vi "Run_Post Core.vi"(0 "For Loop in":refnum<class "While Loop.lvclass">, 11 "error in (no error)":errorcluster) -> (4 "For Loop out":refnum<class "While Loop.lvclass">, 6 "Go to Run Pre Core?":bool, 15 "error out":errorcluster)   [LabVIEW 2016, in "While Loop.lvclass"]
uses:
  While Loop.lvclass
  While Loop.lvclass/While Loop.ctl
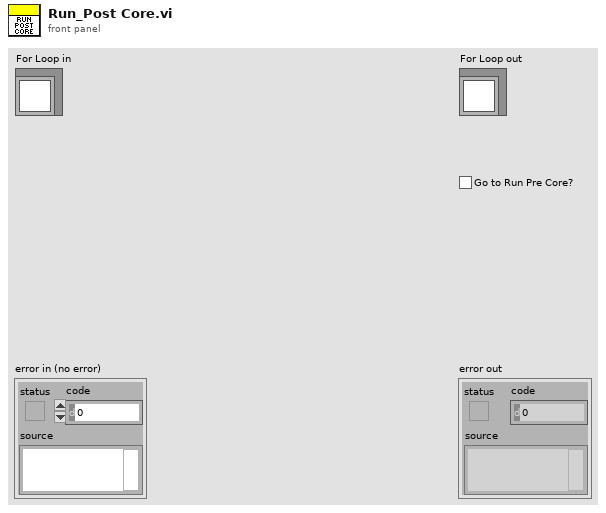
[diagram p1: front panel]
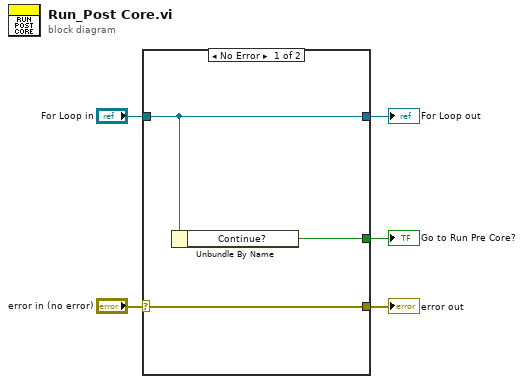
[diagram p0: block diagram]
diagram:
  n1 = case shown="No Error" "error in (no error)" {
    selector: "error in (no error)" -> [w7 w10]
    tunnel: "For Loop in" -> [w6 w9]
    tunnel: [w7 w10] -> w4
    tunnel: [w6 w9] -> w2
    tunnel: [w8 _] -> w1
    frame No Error {
      n2 = Unbundle By Name(w6) -> ("Continue?"=w8:bool)
    }
    frame Error {
    }
  }
  "error out" <- w4
  "For Loop out" <- w2
  "Go to Run Pre Core?" <- w1
